vi "Serial Initialize.vi"(0 "VISA Session In":refnum<visa-resource-name>="OXYMAT", 11 "error in (no error)":errorcluster) -> (4 "VISA Session Out":refnum<visa-resource-name>, 15 "error out":errorcluster)   [LabVIEW 2023, in "Siemens ELAN.lvlib"]
doc: "Lower-level VI which configures the specified VISA session for compatibility with the Siemens ELAN protocol.\n\n$Revision:: 0 $\n$Modtime:: yy-mm-dd hh:mm $\n$Author:: Dboyd $"
uses:
  Siemens ELAN.lvlib
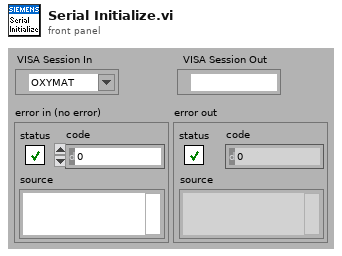
[diagram p1: front panel]
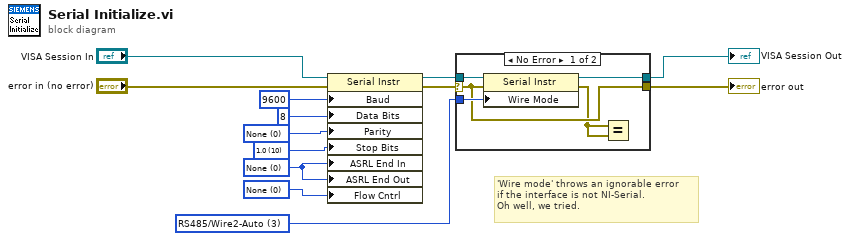
[diagram p0: block diagram]
diagram:
  w5 = i16 3 items=["Unknown"=-1, "RS485/Wire4"=0, "RS485/Wire2-EchoDTR"=1, "RS485/Wire2-CtrlDTR"=2, "RS485/Wire2-Auto"=3, "RS232/DTE"=128, "RS232/DCE"=129, "RS232/AUTO"=130] ("Serial Settings:Wire Mode")
  w8 = u16 0 items=["None", "XON/XOFF", "RTS/CTS", "XON/XOFF & RTS/CTS", "DTR/DSR", "XON/XOFF & DTR/DSR"] ("Serial Settings:Flow Control")
  w9 = u16 0 items=["None", "Last Bit", "TermChar"] ("Serial Settings:End Mode for Reads")
  w10 = u16 10 items=["1.0"=10, "1.5"=15, "2.0"=20] ("Serial Settings:Stop Bits")
  w11 = u16 0 items=["None", "Odd", "Even", "Mark", "Space"] ("Serial Settings:Parity")
  # "'Wire mode' throws an ignorable error\nif the interface is not NI-Serial.\nOh well, we tried."
  n1 = property class="Serial Instr"(reference="VISA Session In", error in="error in (no error)", "Baud"=u32 9600 ("Serial Settings:Baud Rate"), "Data Bits"=u16 8 ("Serial Settings:Data Bits"), "Parity"=w11, "Stop Bits"=w10, "ASRL End In"=w9, "ASRL End Out"=w9, "Flow Cntrl"=w8) -> (reference out=w2:refnum<visa-resource-name>, error out=w4:errorcluster)
  n2 = case shown="No Error" w4 {
    selector: w4 -> [w15 w20]
    tunnel: w5 -> [w18 _]
    tunnel: [w15 w20] -> w3
    tunnel: w2 -> [w17 w19]
    tunnel: [w16 w19] -> w1
    frame No Error {
      n3 = property class="Serial Instr"(reference=w17, error in=w15, "Wire Mode"=w18) -> (reference out=w16:refnum<visa-resource-name>, error out=w14:errorcluster)
      n4 = Equal?(x=w14, y=w14) -> ()  [unwired: 1 out]
    }
    frame Error {
    }
  }
  "VISA Session Out" <- w1
  "error out" <- w3
